vi "PC_Pub_imgFile deployImg.vi"(8 "error in (no error)":errorcluster, 11 "imgFile in":refnum<class "PC_Pub_imgFile.lvclass">) -> (0 "error out":errorcluster, 3 "imgFile out":refnum<class "PC_Pub_imgFile.lvclass">)   [LabVIEW 2018, in "PC_Pub_imgFile.lvclass"]
uses:
  PC_Pub_imgFile.lvclass
  PC_Pub_imgFile.lvclass/PC_Pub_imgFile.ctl
  <vilib>/nisyscfg/nisyscfg.lvlib
  <vilib>/zip/NI_Unzip.lvlib
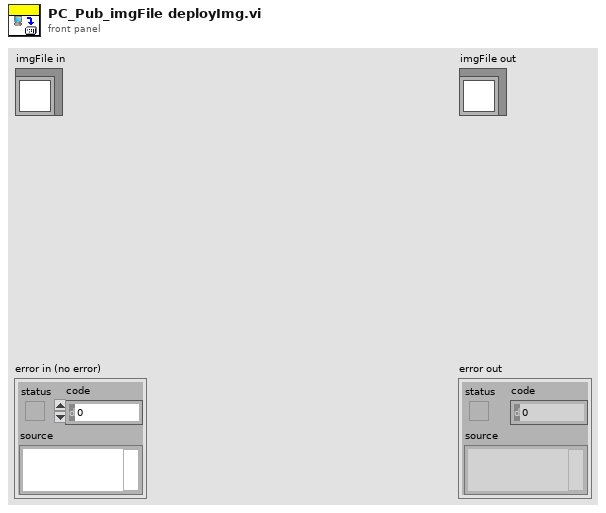
[diagram p1: front panel]
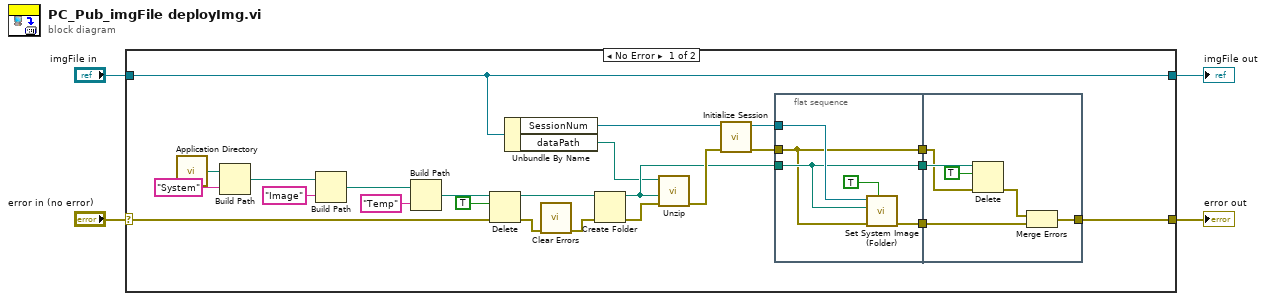
[diagram p0: block diagram]
diagram:
  n1 = case shown="No Error" "error in (no error)" {
    selector: "error in (no error)" -> [w13 w41]
    tunnel: [w6 w41] -> w3
    tunnel: [w28 w40] -> w1
    tunnel: "imgFile in" -> [w28 w40]
    frame No Error {
      n2 = call <vilib>:"Application Directory.vi"() -> ("Application Directory"=w25:path)
      n3 = Build Path(base path=w25, name or relative path="System") -> (appended path=w26:path)
      n4 = Build Path(base path=w26, name or relative path="Image") -> (appended path=w20:path)
      n5 = Build Path(base path=w20, name or relative path="Temp") -> (appended path=w18:path)
      n6 = Delete(path (use dialog)=w18, entire hierarchy (F)=TRUE, error in=w13) -> (deleted path=w21:path, error out=w16:errorcluster)  [unwired: 2 in, 1 out]
      n7 = Unbundle By Name(w28) -> ("SessionNum"=w27:refnum<k21>, "dataPath"=w5:path)
      n8 = call <vilib>:"Clear Errors.vi"("error in (no error)"=w16) -> ("error out"=w15:errorcluster)  [unwired: 5 in, 1 out]
      n9 = Create Folder(path (use dialog)=w21, error in=w15) -> (created path=w10:path, error out=w17:errorcluster)  [unwired: 1 in, 1 out]
      n10 = call <vilib>:"Unzip.vi"("error in (no error)"=w17, "Target directory (same as Zip file if empty)"=w10, "Zip file"=w5) -> ("error out"=w14:errorcluster)  [unwired: 1 in, 7 out]
      n11 = call <vilib>:"Initialize Session.vi"("error in (no error)"=w14, "Target (localhost)"=w27) -> ("error out"=w11:errorcluster, "Session out"=w7:refnum<k21>)  [unwired: 8 in]
      n12 = flat-sequence {
        tunnel: [w32] -> w12
        tunnel: w11 -> [w29]
        tunnel: w7 -> [w31]
        tunnel: w10 -> [w30]
        tunnel: [w30] -> w9
        tunnel: [w29] -> w8
        tunnel: w12 -> [w38]
        tunnel: [w37] -> w6
        tunnel: w9 -> [w36]
        tunnel: w8 -> [w35]
        frame #0 {
          n13 = call <vilib>:"Set System Image (Folder).vi"("Restart Automatically (T)"=TRUE, "error in (no error)"=w29, "Source Folder"=w30, "Session in"=w31) -> ("error out"=w32:errorcluster)  [unwired: 6 in, 1 out]
        }
        frame #1 {
          n14 = Delete(path (use dialog)=w36, entire hierarchy (F)=TRUE, error in=w35) -> (error out=w39:errorcluster)  [unwired: 2 in, 2 out]
          n15 = Merge Errors(w39, w38) -> (w37:errorcluster)
        }
      }
    }
    frame Error {
    }
  }
  "error out" <- w3
  "imgFile out" <- w1
